vi "Initialize Server State.vi"(8 "error in (no error)":errorcluster, 10 "Initial State":T1, 11 "OOP Query Server in":refnum<class "OOP Query Server.lvclass">) -> (0 "error out":errorcluster, 3 "OOP Query Server out":refnum<class "OOP Query Server.lvclass">)   [LabVIEW 2019, in "OOP Query Server.lvlib" / "OOP Query Server.lvclass"]
uses:
  OOP Query Server.lvclass
  typeDefs/Server State Data.ctl
  OOP Query Server.lvclass/OOP Query Server.ctl
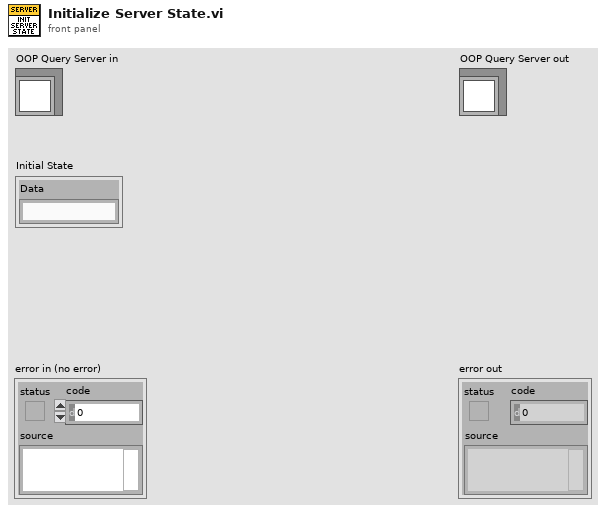
[diagram p1: front panel]
types:
  T1 = typedef "OOP Query Server.lvlib/OOP Query Server.lvclass/Server State Data.ctl" = cluster{"Data":string}
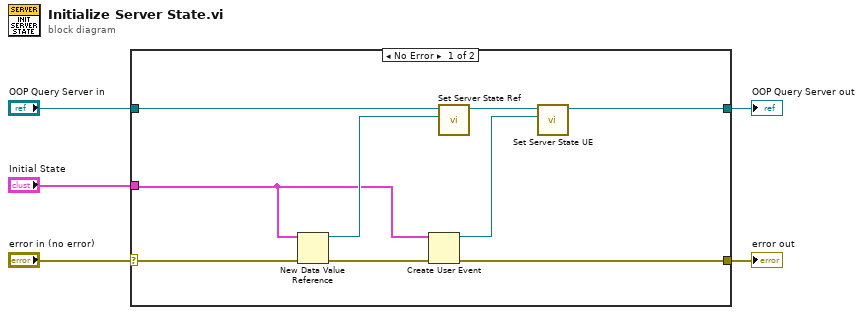
[diagram p0: block diagram]
diagram:
  n1 = case shown="No Error" "error in (no error)" {
    selector: "error in (no error)" -> [w14 w16]
    tunnel: [w12 w16] -> w4
    tunnel: [w7 w15] -> w2
    tunnel: "OOP Query Server in" -> [w11 w15]
    tunnel: "Initial State" -> [w6 _]
    frame No Error {
      n2 = New Data Value Reference(data value=w6, error in=w14) -> (data value reference=w9:refnum<data-value>, error out=w13:errorcluster)
      n3 = Create User Event(user event datatype=w6, error in=w13) -> (user event=w8:refnum<user-event>, error out=w12:errorcluster)
      n4 = call "Set Server State Ref.vi"("Server State Ref"=w9, "OOP Query Server in"=w11) -> ("OOP Query Server out"=w10:refnum<class "OOP Query Server.lvclass">)  [unwired: 9 in]
      n5 = call "Set Server State UE.vi"("Server State UE"=w8, "OOP Query Server in"=w10) -> ("OOP Query Server out"=w7:refnum<class "OOP Query Server.lvclass">)  [unwired: 9 in]
    }
    frame Error {
    }
  }
  "error out" <- w4
  "OOP Query Server out" <- w2
